vi "Create UI.vi"() -> ()   [LabVIEW 2025]
uses:
  Types/Related CAN Frames.ctl
  Types/Base Frame Info.ctl
  <vilib>/NI VeriStand/Custom Device API/Custom Device Item Ref.ctl
  Types/Related CAN Frames No VS.ctl
  Types/Base Frame Info_NoVS.ctl
  <vilib>/Utility/cursorutil.llb/Set Cursor (Icon Pict).vi
  Protection and Counter Addon System Explorer.lvlib
  <vilib>/NI VeriStand/Custom Device API/Custom Device API.lvlib
panel:
  out "Cancel Out":bool
  in  "Cancel":bool
  in  "Update":bool
  in  "Tree":string(tree)
  in  "Changed":T1[](array[typedef])=[{"Old"={"Name"="", "ID"=0, "Signals"=["Same"], "Node Ref"=0}, "Change"={"New"={"Name"="Test", "ID"=0, "Signals"=["New", "Same"]}, "Old"={"Name"="Test", "ID"=1, "Signals"=["Old", "Old1", "Same"]}}}] {"Old"."Node Ref" format="%.0x"}
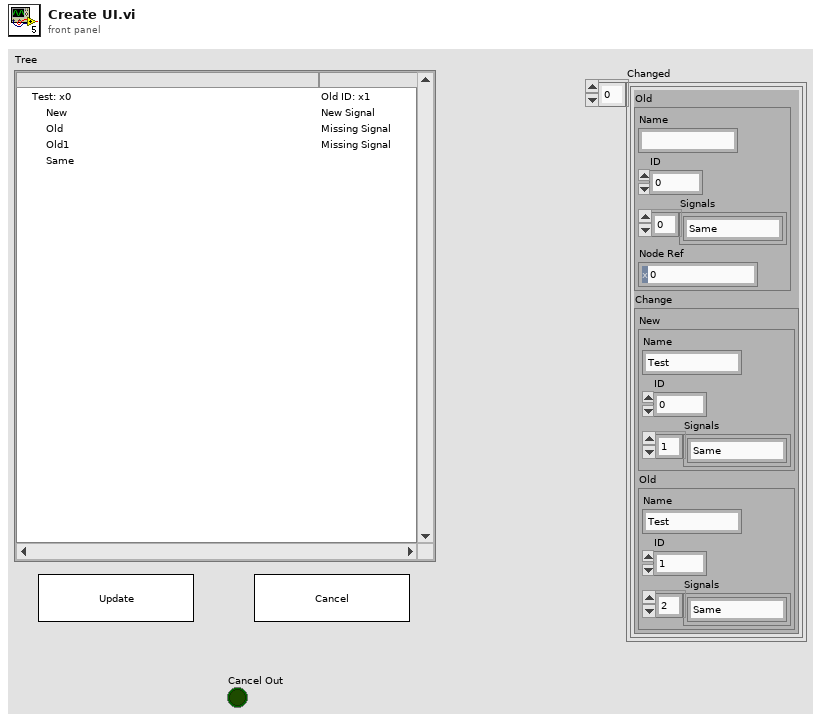
[diagram p1: front panel]
types:
  T1 = typedef "Related CAN Frames.ctl" = cluster{"Old":T2, "Change":T4}
  T2 = typedef "Base Frame Info.ctl" = cluster{"Name":string, "ID":u32, "Signals":string[], "Node Ref":T3}
  T3 = typedef "Custom Device API.lvlib/Custom Device Item Ref.ctl" = u64
  T4 = typedef "Related CAN Frames No VS.ctl" = cluster{"New":T5, "Old":T5}
  T5 = typedef "Base Frame Info_NoVS.ctl" = cluster{"Name":string, "ID":u32, "Signals":string[]}
  T6 = cluster{"Name":string, u32, "Active Item:Symbol Index":i32, "string":string, bool}
  T7 = cluster{"Name":string, u32, "Active Item:Symbol Index":i32, string, bool}
  T8 = cluster{"Name":string, u32, "Active Item:Symbol Index":i32, "string":string, bool}[]
  T9 = typedef "LVPoint32TypeDef.ctl" = cluster{"Horizontal":i32, "Vertical":i32}
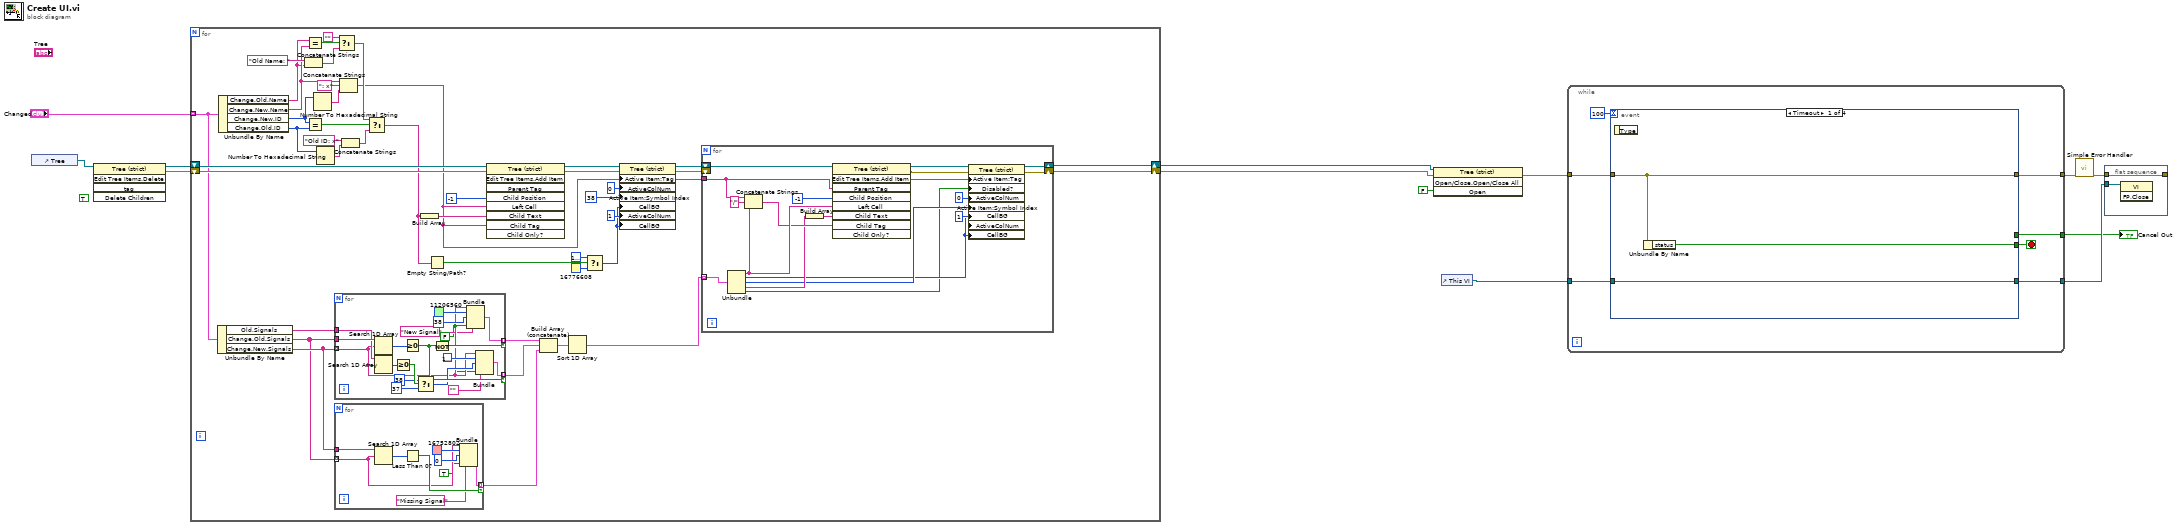
[diagram p0: block diagram]
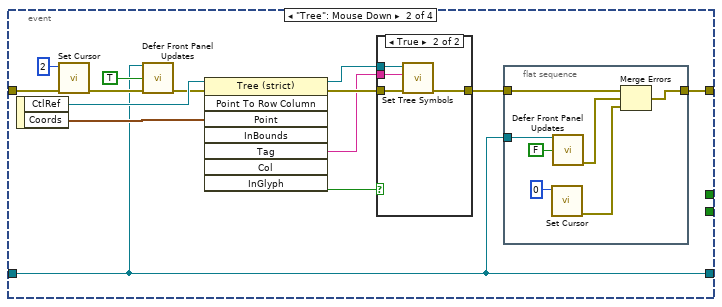
[diagram p2: hidden frame]
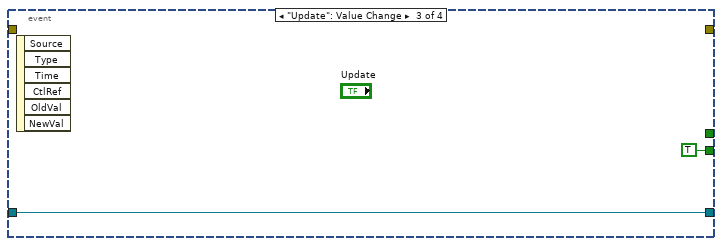
[diagram p4: hidden frame]
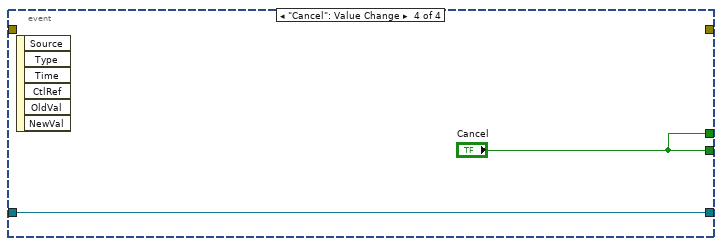
[diagram p5: hidden frame]
diagram:
  (unwired) TRUE ("Delete Children?")
  n1 = control-ref of="Tree"() -> (w13:refnum<vi>)
  n2 = invoke on="Invoke Node" class="Tree (strict)" method="Edit Tree Items.Delete"(reference=w13) -> (reference out=w12:refnum<vi>, error out=w9:errorcluster)  [unwired: 4 in, 3 out]
  n3 = for {
    tunnel: "Changed" -> [w27] mode=indexing
    shift-right: [w15] -> w8
    shift-left: w9 -> [w37]
    shift-right: [w14] -> w7
    shift-left: w12 -> [w53]
    n4 = Unbundle By Name(w27) -> ("Old.Signals"=w24:string[], "Change.Old.Signals"=w25:string[], "Change.New.Signals"=w26:string[])
    n5 = Unbundle By Name(w27) -> ("Change.Old.Name"=w43:string, "Change.New.Name"=w47:string, "Change.New.ID"=w45:u32, "Change.Old.ID"=w49:u32)
    n6 = Concatenate Strings("Old Name: ", w43) -> (w38:string)
    n7 = Equal?(x=w43, y=w47) -> (x = y?=w39:bool)
    n8 = Equal?(x=w45, y=w49) -> (x = y?=w42:bool)
    n9 = Number To Hexadecimal String(2:w45) -> (0:w44:string)  [unwired: 1 in]
    n10 = Number To Hexadecimal String(2:w49) -> (0:w48:string)  [unwired: 1 in]
    n11 = for {
      tunnel: w25 -> [w103]
      tunnel: w26 -> [w88] mode=indexing
      tunnel: [w90] -> w22 mode=indexing if=w101
      tunnel: [w89] -> w23 mode=indexing if=w100
      tunnel: w24 -> [w96]
      w85 = FALSE
      n12 = Search 1D Array(1D array=w103, element=w88) -> (index of element=w102:i32)  [unwired: 1 in]
      n13 = Search 1D Array(1D array=w96, element=w88) -> (index of element=w95:i32)  [unwired: 1 in]
      n14 = Greater Or Equal To 0?(x=w95) -> (x >= 0?=w94:bool)
      n15 = Greater Or Equal To 0?(x=w102) -> (x >= 0?=w101:bool)
      n16 = Select(t=38 ("Active Item:Symbol Index"), s=w94, f=37 ("Active Item:Symbol Index")) -> (s? t:f=w91:i32)
      n17 = Not(x=w101) -> (.not. x?=w100:bool)
      n18 = Bundle("Name"=w88, u32 11206560, "Active Item:Symbol Index"=38, "string"="New Signal", w85) -> (w89:T6)  [unwired: 1 in]
      n19 = Bundle("Name"=w88, u32 16777216, "Active Item:Symbol Index"=w91, "", w85) -> (w90:T7)  [unwired: 1 in]
    }
    n20 = for {
      tunnel: w26 -> [w84]
      tunnel: w25 -> [w78] mode=indexing
      tunnel: [w79] -> w21 mode=indexing if=w82
      n21 = Search 1D Array(1D array=w84, element=w78) -> (index of element=w83:i32)  [unwired: 1 in]
      n22 = Less Than 0?(x=w83) -> (x < 0?=w82:bool)
      n23 = Bundle("Name"=w78, u32 16752802, "Active Item:Symbol Index"=0, "string"="Missing Signal", TRUE) -> (w79:T6)  [unwired: 1 in]
    }
    n24 = Select(t="", s=w39, f=w38) -> (s? t:f=w35:string)
    n25 = Concatenate Strings(w47, ": x" ("string"), w44) -> (w16:string)
    n26 = Concatenate Strings("Old ID: x", w48) -> (w41:string)
    n27 = Select(t=w35, s=w42, f=w41) -> (s? t:f=w34:string)
    n28 = Build Array(w34) -> (w36:string[])
    n29 = Empty String/Path?(string/path=w34) -> (empty?=w33:bool)
    n30 = invoke on="Invoke Node" class="Tree (strict)" method="Edit Tree Items.Add Item"(reference=w53, error in=w37, "Child Position"=-1, "Left Cell"=w16, "Child Text"=w36, "Child Tag"=w16) -> (reference out=w56:refnum<vi>, error out=w55:errorcluster)  [unwired: 3 in, 7 out]
    n31 = Build Array (concatenate)(w23, w22, w21) -> (w20:T8)
    n32 = Sort 1D Array(array=w20) -> (sorted array=w17:T8)
    n33 = Select(t=u32 16777216, s=w33, f=u32 16776608) -> (s? t:f=w28:u32)
    n34 = property class="Tree (strict)"(reference=w56, error in=w55, "Active Item:Tag"=w16, "ActiveColNum"=0 ("Active Cell:Active Column Number"), "Active Item:Symbol Index"=38, "CellBG"=w28, "ActiveColNum"=1 ("Active Cell:Active Column Number"), "CellBG"=w28) -> (reference out=w19:refnum<vi>, error out=w18:errorcluster)
    n35 = for {
      shift-right: [w58] -> w14
      shift-left: w19 -> [w73]
      shift-right: [w59] -> w15
      shift-left: w18 -> [_]
      tunnel: w17 -> [w71] mode=indexing
      tunnel: w16 -> [w72]
      n36 = Unbundle(w71) -> ("Name"=w70:string, w60:u32, "Active Item:Symbol Index"=w61:i32, "string"=w68:string, w57:bool)
      n37 = Concatenate Strings(w72, "/" ("string"), w70) -> (w69:string)
      n38 = Build Array(w68) -> (w67:string[])
      n39 = invoke on="Invoke Node" class="Tree (strict)" method="Edit Tree Items.Add Item"(reference=w73, "Parent Tag"=w72, "Child Position"=-1, "Left Cell"=w70, "Child Text"=w67, "Child Tag"=w69) -> (reference out=w64:refnum<vi>, error out=w63:errorcluster, "Edit Tree Items:Add Item"=w62:string)  [unwired: 3 in, 6 out]
      n40 = property class="Tree (strict)"(reference=w64, error in=w63, "Active Item:Tag"=w62, "Disabled?"=w57, "ActiveColNum"=0 ("Active Cell:Active Column Number"), "Active Item:Symbol Index"=w61, "CellBG"=w60, "ActiveColNum"=1 ("Active Cell:Active Column Number"), "CellBG"=w60) -> (reference out=w58:refnum<vi>, error out=w59:errorcluster)
    }
  }
  n41 = invoke on="Invoke Node" class="Tree (strict)" method="Open/Close.Open/Close All"(reference=w7, error in=w8, "Open"=FALSE ("Open?")) -> (error out=w6:errorcluster)  [unwired: 1 in, 3 out]
  n42 = control-ref of="This VI"() -> (w5:refnum<vi>)
  n43 = while {
    tunnel: w6 -> [w110]
    tunnel: w5 -> [w109]
    tunnel: [w107] -> w3
    tunnel: [w106] -> w2
    tunnel: [w105] -> w1
    stop <- w108 stop-if-true
    n44 = event shown="[0] Timeout" {
      selector: _ -> [_ _ _ _]
      dyn-events: _ -> [_ _ _ _]
      timeout: 100 -> [_ _ _ _]
      tunnel: w110 -> [w113 w120 _ _]
      tunnel: [w112 _ TRUE ("status") "Cancel"] -> w108
      tunnel: [w113 w118 _ _] -> w107
      tunnel: w109 -> [w111 w114 w140 w143]
      tunnel: [w111 w114 w140 w143] -> w106
      tunnel: [_ _ _ "Cancel"] -> w105
      event Timeout {
        n45 = event-data() -> ()  [unwired: 1 in, 1 out]
        n46 = Unbundle By Name(w113) -> ("status"=w112:bool)
      }
      event "Tree": Mouse Down {
        n47 = event-data() -> ("CtlRef"=w126:refnum<vi>, "Coords"=w127:T9)  [unwired: 1 in]
        n48 = call-poly <vilib>:"Set Cursor.vi"("error in (no error)"=w120, "icon"=u16 2) -> ("error out"=w116:errorcluster)  [unwired: 8 in, 1 out]
        n49 = call "Defer Front Panel Updates.vi"("This VI"=w114, "Defer Panel Updates"=TRUE, "error in (no error)"=w116) -> ("error out"=w115:errorcluster)  [unwired: 12 in]
        n50 = invoke on="Invoke Node" class="Tree (strict)" method="Point To Row Column"(reference=w126, error in=w115, "Point"=w127) -> (reference out=w124:refnum<vi>, error out=w125:errorcluster, "Tag"=w123:string, "InGlyph"=w122:bool)  [unwired: 5 in, 4 out]
        n51 = case shown="True" w122 {
          tunnel: w125 -> [w135 w139]
          tunnel: w124 -> [_ w138]
          tunnel: w123 -> [_ w137]
          tunnel: [w135 w136] -> w119
          frame False {
          }
          frame True {
            n52 = call "Set Tree Symbols.vi"("error in"=w139, "Tag"=w137, "CtlRef"=w138) -> ("error out"=w136:errorcluster)  [unwired: 8 in]
          }
        }
        n53 = flat-sequence {
          tunnel: [w131] -> w118
          tunnel: w119 -> [w132]
          tunnel: w114 -> [w128]
          frame #0 {
            n54 = call-poly <vilib>:"Set Cursor.vi"("icon"=u16 0) -> ("error out"=w133:errorcluster)  [unwired: 9 in, 1 out]
            n55 = call "Defer Front Panel Updates.vi"("This VI"=w128, "Defer Panel Updates"=FALSE) -> ("error out"=w129:errorcluster)  [unwired: 13 in]
            n56 = Merge Errors(w132, w129, w133) -> (w131:errorcluster)
          }
        }
      }
      event "Update": Value Change {
        n57 = event-data() -> ()  [unwired: 1 in, 6 out]
      }
      event "Cancel": Value Change {
        n58 = event-data() -> ()  [unwired: 1 in, 6 out]
      }
    }
  }
  "Cancel Out" <- w1
  n59 = call <vilib>:"Simple Error Handler.vi"("error in (no error)"=w3) -> ("error out"=w4:errorcluster)  [unwired: 4 in, 4 out]
  n60 = flat-sequence {
    tunnel: [w145] -> _
    tunnel: w4 -> [w145]
    tunnel: w2 -> [w144]
    frame #0 {
      n61 = invoke class="VI" method="FP.Close"(reference=w144) -> ()  [unwired: 2 in, 3 out]
    }
  }
